vi "Read Mode Select.vi"(8 "error in (no error)":errorcluster, 11 "Task Data in":refnum<class "Task Data.lvclass">) -> (0 "error out":errorcluster, 2 "Mode Select":T1, 3 "Task Data out":refnum<class "Task Data.lvclass">)   [LabVIEW 2012, in "Task Data.lvclass"]
uses:
  Task Data.lvclass
  Type Defs/Mode Select.ctl
  Task Data.lvclass/Task Data.ctl
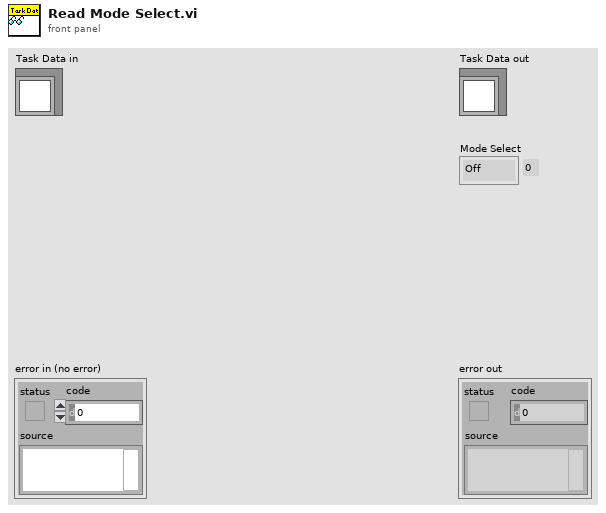
[diagram p1: front panel]
types:
  T1 = typedef "Mode Select.ctl" = enum8{"Off", "Stby", "Hold", "Run"}
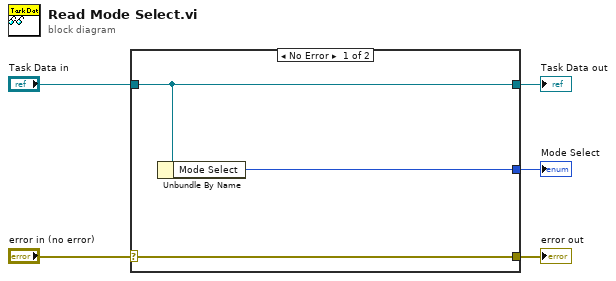
[diagram p0: block diagram]
diagram:
  n1 = case shown="No Error" "error in (no error)" {
    selector: "error in (no error)" -> [w8 w9]
    tunnel: [w8 w9] -> w4
    tunnel: [w7 w10] -> w2
    tunnel: "Task Data in" -> [w7 w10]
    tunnel: [w6 _] -> w1
    frame No Error {
      n2 = Unbundle By Name(w7) -> ("Mode Select"=w6:T1)
    }
    frame Error {
    }
  }
  "error out" <- w4
  "Task Data out" <- w2
  "Mode Select" <- w1
